vi "ex3.vi"() -> ()   [LabVIEW 2018]
uses:
  <vilib>/Analysis/3filter.llb/Filter Passband Type.ctl
  <vilib>/Analysis/2dsp.llb/Real FFT.vi
  <vilib>/Analysis/3filter.llb/Butterworth Filter (DBL).vi
  <vilib>/measure/matone.llb/Extract Single Tone Information 1 Chan.vi
  <vilib>/Waveform/WDTOps.llb/WDT Append Waveforms DBL.vi
  <vilib>/Waveform/WDTOps.llb/WDT Waveform Duration DBL.vi
  <vilib>/Waveform/WDTFileIO.llb/Export Waveform To Spreadsheet File.vi
  <vilib>/Analysis/NI_AALPro.lvlib
  <vilib>/measure/NI_MAPro.lvlib
  <vilib>/Analysis/NI_AALBase.lvlib
panel:
  out "x-y":dbl
  out "Phase":dbl
  out "detected phase (deg)":dbl format="%.2p"
  out "Waveform Graph 5":dbl[](graph)
  out "arctan(x)":dbl
  out "Numeric 5":dbl format="%#_13g"
  out "Numeric 4":dbl format="%#_13g"
  out "Numeric 3":dbl format="%#_13g"
  out "x >= y? 3":bool
  out "x >= y? 2":bool
  out "x >= y?":bool
  out "duration":dbl format="%0.2f"
  out "size(s)":i32
  out "Numeric 2":dbl format="%#_13g"
  out "Numeric":dbl
  out "Array 4":dbl[](array[numeric])
  out "Array 3":dbl[](array[numeric])
  out "Array 2":dbl[](array[numeric])
  out "Array":dbl[](array[numeric])
  out "Waveform Graph 4":dynamicdata(graph)
  out "Waveform Graph 3":dynamicdata(graph)
  out "Waveform Graph 2":dynamicdata(graph)
  out "Waveform Graph":dynamicdata(graph)
  in  "stop (F)":bool
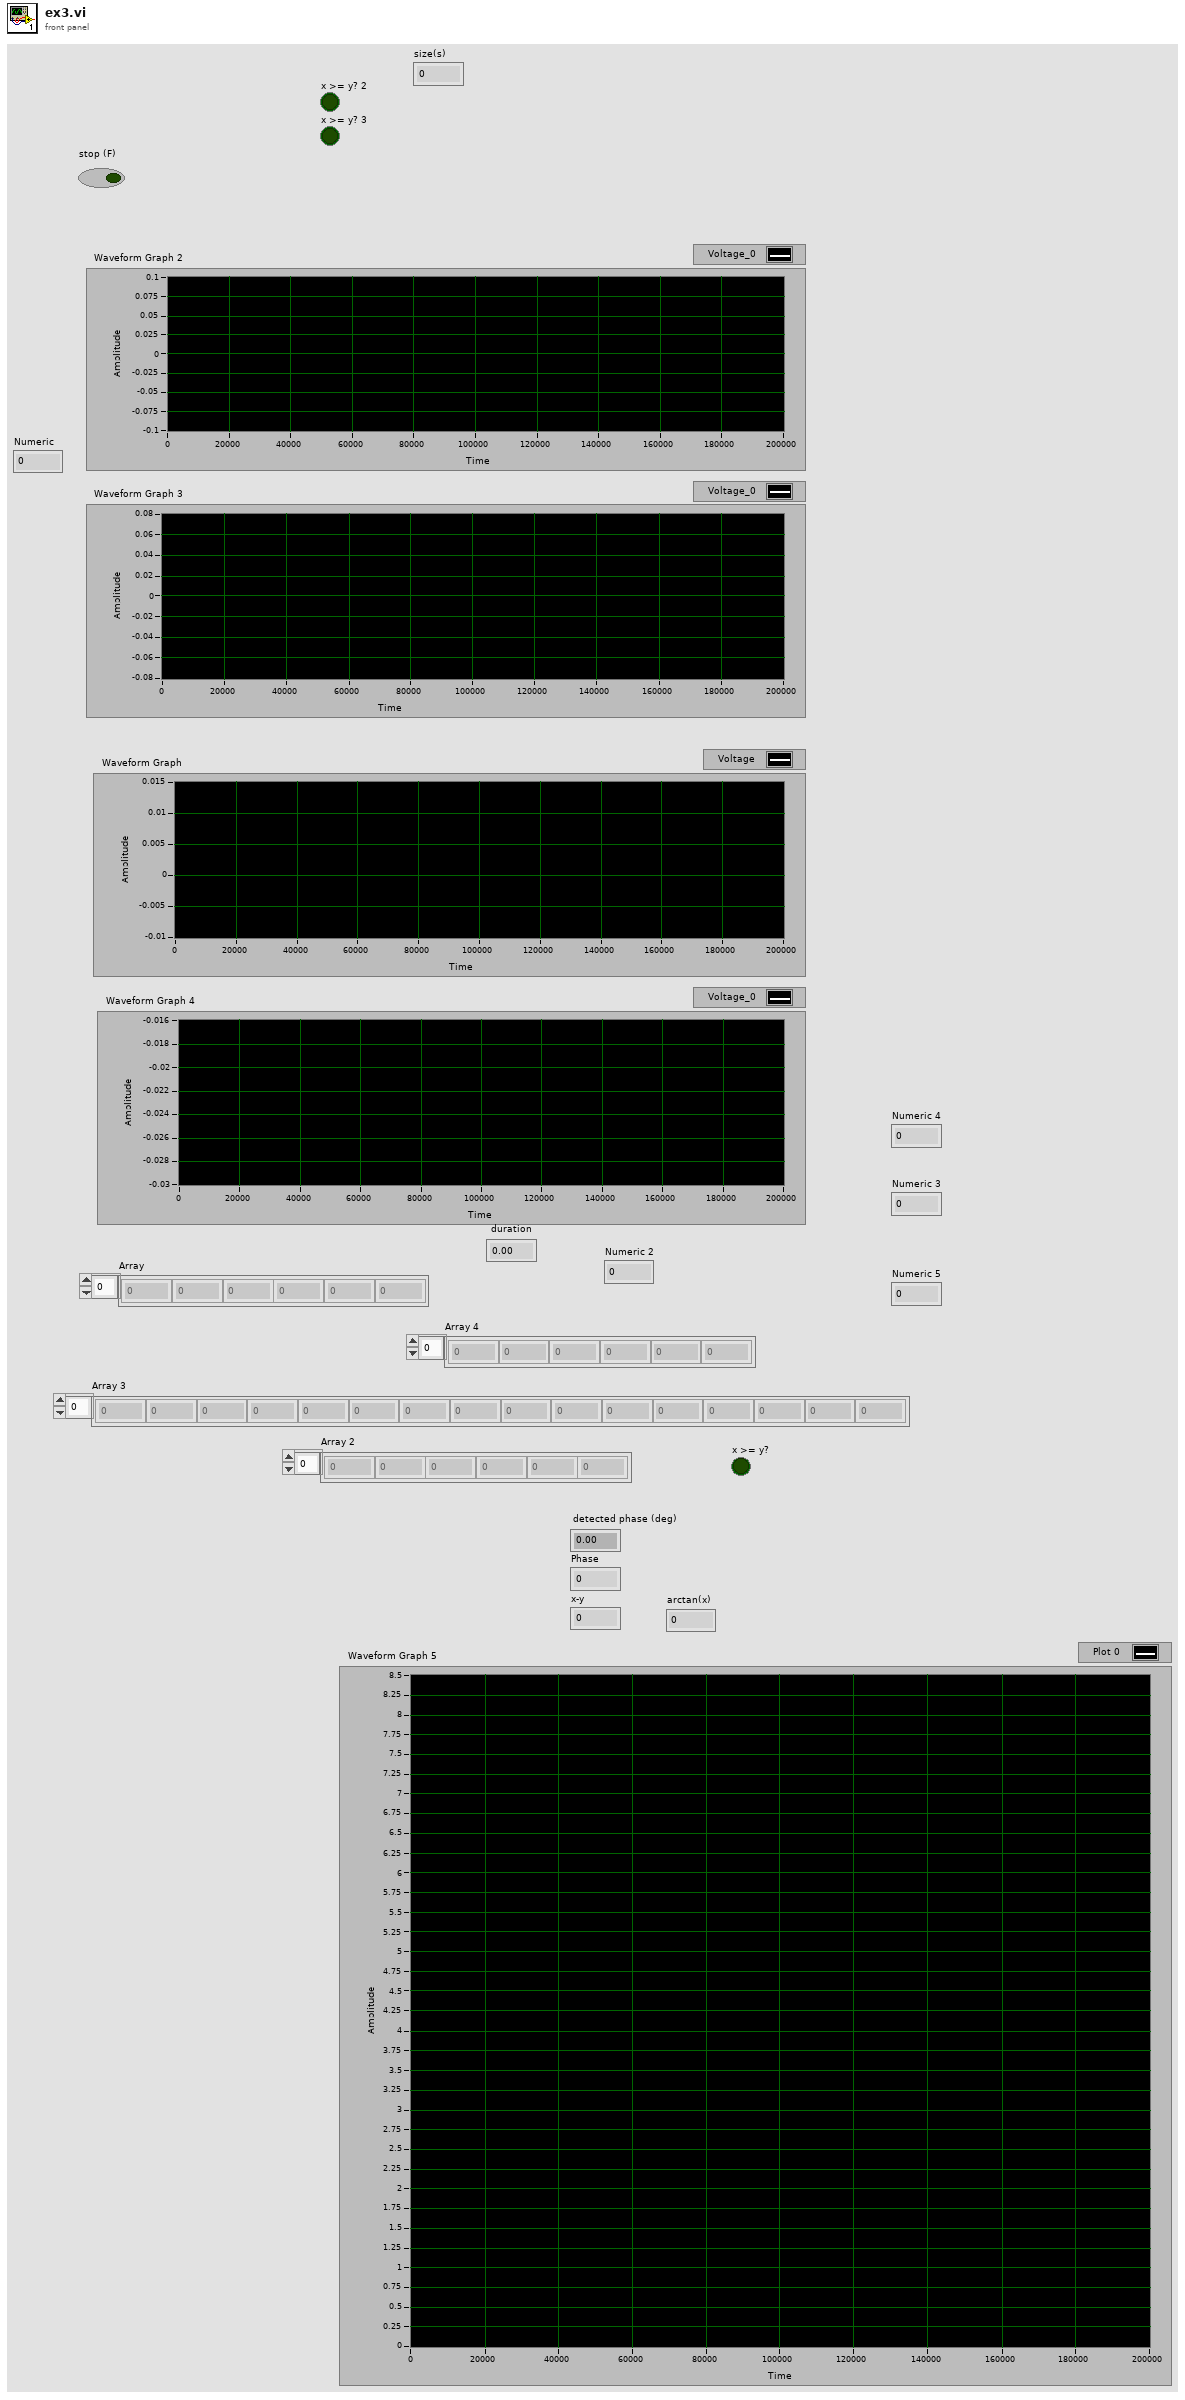
[diagram p1: front panel]
types:
  T1 = typedef "NI_AALBase.lvlib/Filter Passband Type.ctl" = enum32{"Lowpass", "Highpass", "Bandpass", "Bandstop"}
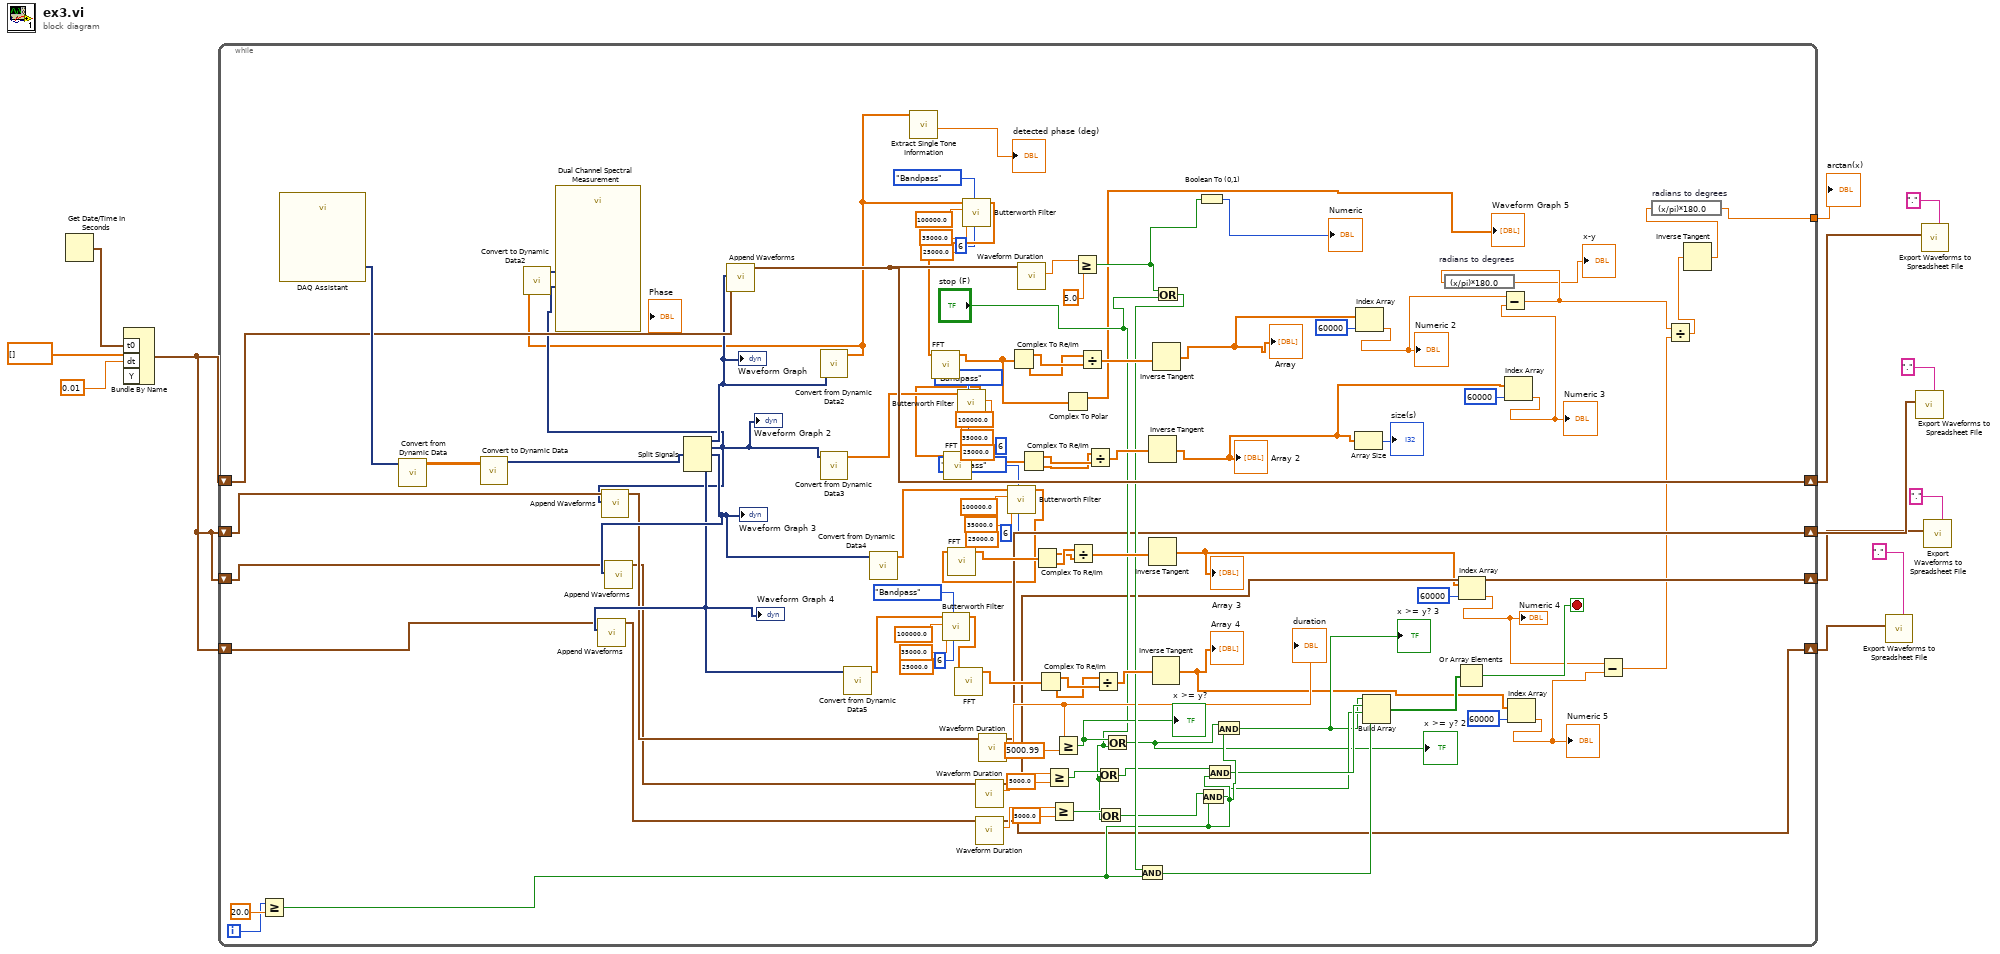
[diagram p0: block diagram]
diagram:
  n1 = Get Date/Time In Seconds() -> (seconds since 1Jan1904=w13:timestamp)
  n2 = Bundle By Name("t0"=w13, "dt"=0.01, "Y"=dbl[] []) -> (w10:waveform(dbl))  [unwired: 1 in]
  n3 = while {
    shift-right: [w106] -> w9
    shift-left: w10 -> [w108]
    shift-right: [w73] -> w8
    shift-left: w10 -> [w76]
    shift-right: [w72] -> w7
    shift-left: w10 -> [w75]
    shift-right: [w71] -> w6
    shift-left: w10 -> [w74]
    tunnel: [w40] -> w1
    i -> [w102]
    stop <- w77 stop-if-true
    (unwired) 25000.0 ("low cutoff freq: fl")
    (unwired) 25000.0 ("low cutoff freq: fl")
    (unwired) 25000.0 ("low cutoff freq: fl")
    n4 = Greater Or Equal?(x=w102, y=20.0) -> (x >= y?=w82:bool)
    n5 = call "DAQ Assistant"() -> ("data"=w114:dynamicdata)  [unwired: 16 in, 3 out]
    n6 = call "Convert from Dynamic Data"("Dynamic Data Type"=w114) -> ("Array"=w113:dbl[][])  [unwired: 3 in]
    n7 = call "Convert to Dynamic Data"("2D Array"=w113) -> ("Dynamic Data Type"=w107:dynamicdata)  [unwired: 3 in]
    n8 = Split Signals(w107) -> (w100:dynamicdata, w41:dynamicdata, w99:dynamicdata, w98:dynamicdata)  [unwired: 5 in, 1 out]
    "Waveform Graph" <- w100
    "Waveform Graph 2" <- w41
    "Waveform Graph 3" <- w99
    "Waveform Graph 4" <- w98
    n9 = call-poly <vilib>:"Append Waveforms.vi"("waveform B"=w98, "waveform A"=w74) -> ("waveform out"=w95:waveform(dbl))  [unwired: 8 in, 1 out]
    n10 = call-poly <vilib>:"Append Waveforms.vi"("waveform B"=w41, "waveform A"=w76) -> ("waveform out"=w97:waveform(dbl))  [unwired: 8 in, 1 out]
    n11 = call-poly <vilib>:"Append Waveforms.vi"("waveform B"=w99, "waveform A"=w75) -> ("waveform out"=w96:waveform(dbl))  [unwired: 8 in, 1 out]
    n12 = call-poly <vilib>:"Append Waveforms.vi"("waveform B"=w100, "waveform A"=w108) -> ("waveform out"=w106:waveform(dbl))  [unwired: 8 in, 1 out]
    n13 = call "Convert from Dynamic Data2"("Dynamic Data Type"=w100) -> ("Array"=w39:dbl[])  [unwired: 3 in]
    n14 = call "Convert to Dynamic Data2"("Array"=w39) -> ("Dynamic Data Type"=w44:dynamicdata)  [unwired: 3 in]
    n15 = call "Dual Channel Spectral Measurement"("Input Signal B"=w41, "Input Signal A"=w44) -> ()  [unwired: 7 in, 3 out]
    n16 = call "Convert from Dynamic Data3"("Dynamic Data Type"=w41) -> ("Array"=w15:dbl[])  [unwired: 3 in]
    n17 = call "Convert from Dynamic Data5"("Dynamic Data Type"=w98) -> ("Array"=w19:dbl[])  [unwired: 3 in]
    n18 = call "Convert from Dynamic Data4"("Dynamic Data Type"=w99) -> ("Array"=w17:dbl[])  [unwired: 3 in]
    n19 = call-poly <vilib>:"Extract Single Tone Information.vi"("time signal in"=w39) -> ("detected phase (deg)"=→"detected phase (deg)":dbl)  [unwired: 5 in, 5 out]
    n20 = call-poly <vilib>:"Butterworth Filter.vi"("order"=6, "filter type"=Filter_Passband_Type."Bandpass", "high cutoff freq: fh"=35000.0, "sampling freq: fs"=100000.0, "X"=w19) -> ("Filtered X"=w18:dbl[])  [unwired: 3 in, 1 out]
    n21 = call-poly <vilib>:"FFT.vi"("X"=w18) -> ("FFT {X}"=w119:cdb[])  [unwired: 9 in, 1 out]
    n22 = call-poly <vilib>:"Butterworth Filter.vi"("order"=6, "filter type"=Filter_Passband_Type."Bandpass", "high cutoff freq: fh"=35000.0, "sampling freq: fs"=100000.0, "X"=w15) -> ("Filtered X"=w14:dbl[])  [unwired: 3 in, 1 out]
    n23 = call-poly <vilib>:"FFT.vi"("X"=w14) -> ("FFT {X}"=w121:cdb[])  [unwired: 9 in, 1 out]
    n24 = call-poly <vilib>:"Butterworth Filter.vi"("order"=6, "filter type"=Filter_Passband_Type."Bandpass", "low cutoff freq: fl"=25000.0, "high cutoff freq: fh"=35000.0, "sampling freq: fs"=100000.0, "X"=w39) -> ("Filtered X"=w38:dbl[])  [unwired: 2 in, 1 out]
    n25 = call-poly <vilib>:"FFT.vi"("X"=w38) -> ("FFT {X}"=w46:cdb[])  [unwired: 9 in, 1 out]
    n26 = call-poly <vilib>:"Waveform Duration.vi"("waveform in"=w96) -> ("duration"=w92:dbl, "waveform out"=w72:waveform(dbl))  [unwired: 8 in, 1 out]
    n27 = call-poly <vilib>:"Waveform Duration.vi"("waveform in"=w95) -> ("duration"=w90:dbl, "waveform out"=w71:waveform(dbl))  [unwired: 8 in, 1 out]
    n28 = call-poly <vilib>:"Waveform Duration.vi"("waveform in"=w97) -> ("duration"=w94:dbl, "waveform out"=w73:waveform(dbl))  [unwired: 8 in, 1 out]
    "duration" <- w94
    n29 = call-poly <vilib>:"Butterworth Filter.vi"("order"=6, "filter type"=Filter_Passband_Type."Bandpass", "high cutoff freq: fh"=35000.0, "sampling freq: fs"=100000.0, "X"=w17) -> ("Filtered X"=w16:dbl[])  [unwired: 3 in, 1 out]
    n30 = call-poly <vilib>:"FFT.vi"("X"=w16) -> ("FFT {X}"=w120:cdb[])  [unwired: 9 in, 1 out]
    n31 = Complex To Re/Im(x + iy=w46) -> (x=w48:dbl[], y=w47:dbl[])
    n32 = call-poly <vilib>:"Waveform Duration.vi"("waveform in"=w106) -> ("duration"=w111:dbl)  [unwired: 8 in, 2 out]
    n33 = Complex To Re/Im(x + iy=w121) -> (x=w67:dbl[], y=w66:dbl[])
    n34 = Complex To Re/Im(x + iy=w120) -> (x=w64:dbl[], y=w65:dbl[])
    n35 = Complex To Re/Im(x + iy=w119) -> (x=w63:dbl[], y=w62:dbl[])
    n36 = Greater Or Equal?(x=w92, y=5000.0) -> (x >= y?=w87:bool)
    n37 = Greater Or Equal?(x=w90, y=5000.0) -> (x >= y?=w86:bool)
    n38 = Greater Or Equal?(x=w94, y=5000.99) -> (x >= y?=w88:bool)
    "x >= y?" <- w88
    n39 = Complex To Polar(r * e^(i*theta)=w46) -> (r=→"Waveform Graph 5":dbl[])  [unwired: 1 out]
    n40 = Divide(x=w65, y=w64) -> (x/y=w117:dbl[])
    n41 = Greater Or Equal?(x=w111, y=5.0) -> (x >= y?=w110:bool)
    n42 = Divide(x=w47, y=w48) -> (x/y=w115:dbl[])
    n43 = Divide(x=w66, y=w67) -> (x/y=w116:dbl[])
    n44 = Divide(x=w62, y=w63) -> (x/y=w118:dbl[])
    n45 = Or(x=w87, y="stop (F)") -> (x .or. y?=w84:bool)
    n46 = Or(x=w86, y="stop (F)") -> (x .or. y?=w83:bool)
    n47 = Or(x=w88, y="stop (F)") -> (x .or. y?=w69:bool)
    "x >= y? 2" <- w69
    n48 = Inverse Tangent(1:w116) -> (0:w58:dbl[])
    "Array 2" <- w58
    n49 = Inverse Tangent(1:w117) -> (0:w59:dbl[])
    "Array 3" <- w59
    n50 = Inverse Tangent(1:w118) -> (0:w56:dbl[])
    "Array 4" <- w56
    n51 = Inverse Tangent(1:w115) -> (0:w105:dbl[])
    "Array" <- w105
    n52 = Or(x=w110, y="stop (F)") -> (x .or. y?=w101:bool)
    n53 = And(x=w101, y=w82) -> (x .and. y?=w79:bool)
    n54 = Boolean To (0,1)(Boolean=w110) -> (0, 1=→"Numeric":i16)
    n55 = And(x=w83, y=w82) -> (x .and. y?=w80:bool)
    n56 = And(x=w84, y=w82) -> (x .and. y?=w81:bool)
    n57 = And(x=w69, y=w82) -> (x .and. y?=w68:bool)
    "x >= y? 3" <- w68
    n58 = Array Size(array=w58) -> (size(s)=→"size(s)":i32)
    n59 = Index Array(array=w105, index=60000) -> (element=w55:dbl)
    "Numeric 2" <- w55
    n60 = Build Array(w68, w81, w80, w79) -> (w78:bool[])
    n61 = Or Array Elements(Boolean array=w78) -> (logical OR=w77:bool)
    n62 = Index Array(array=w59, index=60000) -> (element=w52:dbl)
    "Numeric 4" <- w52
    n63 = Index Array(array=w58, index=60000) -> (element=w54:dbl)
    "Numeric 3" <- w54
    n64 = Subtract(x=w55, y=w54) -> (x-y=w43:dbl)
    n65 = expression code="(x/pi)*180.0" "radians to degrees"(w43) -> (→"x-y":dbl)
    n66 = Index Array(array=w56, index=60000) -> (element=w53:dbl)
    "Numeric 5" <- w53
    n67 = Subtract(x=w52, y=w53) -> (x-y=w51:dbl)
    n68 = Divide(x=w43, y=w51) -> (x/y=w50:dbl)
    n69 = Inverse Tangent(1:w50) -> (0:w49:dbl)
    n70 = expression code="(x/pi)*180.0" "radians to degrees"(w49) -> (w40:dbl)
  }
  "arctan(x)" <- w1
  n71 = call-poly <vilib>:"Export Waveforms to Spreadsheet File.vi"("delimiter (Tab)"=".", "waveform"=w6) -> ()  [unwired: 8 in, 2 out]
  n72 = call-poly <vilib>:"Export Waveforms to Spreadsheet File.vi"("delimiter (Tab)"=".", "waveform"=w8) -> ()  [unwired: 8 in, 2 out]
  n73 = call-poly <vilib>:"Export Waveforms to Spreadsheet File.vi"("delimiter (Tab)"=".", "waveform"=w9) -> ()  [unwired: 8 in, 2 out]
  n74 = call-poly <vilib>:"Export Waveforms to Spreadsheet File.vi"("delimiter (Tab)"=".", "waveform"=w7) -> ()  [unwired: 8 in, 2 out]
